vi "Create TDM.vi"() -> ()   [LabVIEW 2011]
uses:
  <vilib>/Platform/storage/lvStorage.llb/_openFunction.ctl
  <vilib>/Platform/storage/Storage.llb/usiSequenceRepresentation.ctl
  <vilib>/Platform/storage/lvStorage.llb/_defaultFilePath.vi
  <vilib>/Platform/storage/lvStorage.llb/_openStorageWithRootAutoDetect.vi
  <vilib>/Platform/storage/lvStorage.llb/xStorage/xStorageSupp/ErrorOut.vi
  <vilib>/Platform/storage/lvStorage.llb/_prepDDT.vi
  <vilib>/Platform/storage/lvStorage.llb/_createOrGetExplicitChildObject.vi
  <vilib>/Platform/storage/lvStorage.llb/_getChannelNameFromDDT.vi
  <vilib>/Platform/storage/lvStorage.llb/_createOrGetByNameExplicitChildObject.vi
  <vilib>/Platform/storage/lvStorage.llb/_saveDDT.vi
  <vilib>/Platform/storage/lvStorage.llb/_queryPropDateTime.vi
  <vilib>/Platform/storage/lvStorage.llb/_queryGenericObjects.vi
  <vilib>/Platform/storage/lvStorage.llb/_loadAllDdt.vi
  <vilib>/Platform/storage/Storage.llb/Get Object Info.vi
  <vilib>/Platform/storage/Storage.llb/__closeStorageFromObject.vi
  <vilib>/Platform/storage/lvStorage.llb/xStorage/Open Data Storage/Open Data Storage.xnode
  <vilib>/Platform/storage/lvStorage.llb/xStorage/Write Data/Write Data.xnode
  <vilib>/Platform/storage/lvStorage.llb/xStorage/Read Data/Read Data.xnode
  <vilib>/Platform/storage/lvStorage.llb/xStorage/Close Data Storage/Close Data Storage.xnode
panel:
  out "Waveform Graph":dynamicdata(graph)
  out "error out":errorcluster
  in  "stop":bool
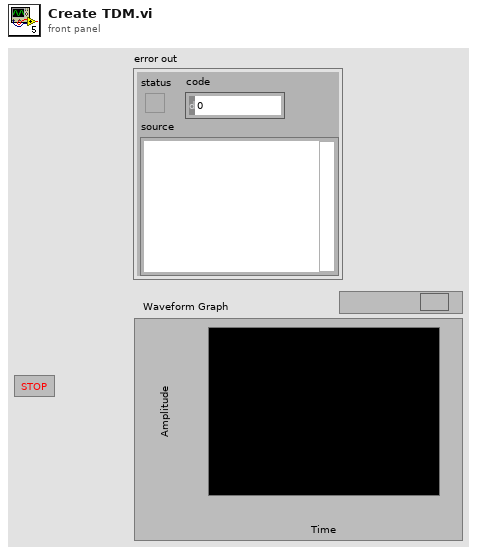
[diagram p1: front panel]
types:
  T1 = enum16{"Append values", "Replace values at index", "Replace all values"}
  T2 = enum16{"UPDATE", "READ", "QUERY", "CREATE CHILD", "CREATE", "CONNECT", "DISCONNECT"}
  T3 = typedef "usiSequenceRepresentation.ctl" = enum16{"explicit", "implicit"}
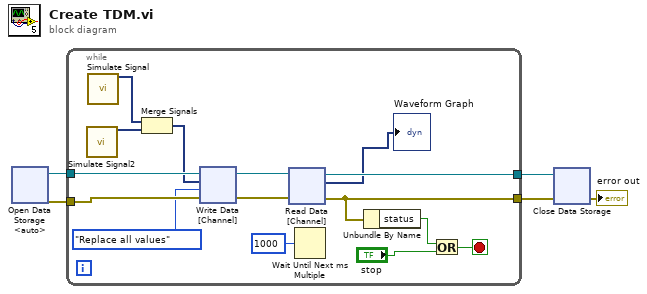
[diagram p0: block diagram]
diagram:
  n1 = xnode "Open Data Storage\n<auto>"() -> ("storage refnum (file)"=w5:refnum<k20>, "error out"=w4:errorcluster)  [unwired: 5 in, 1 out]
  n2 = while {
    tunnel: w5 -> [w20]
    tunnel: w4 -> [w19]
    tunnel: [w10] -> w3
    tunnel: [w11] -> w2
    stop <- w7 stop-if-true
    n3 = call "Simulate Signal2"() -> ("Sawtooth"=w17:dynamicdata)  [unwired: 14 in, 1 out]
    n4 = call "Simulate Signal"() -> ("Sine"=w18:dynamicdata)  [unwired: 14 in, 1 out]
    n5 = Merge Signals(w18, w17) -> (w12:dynamicdata)
    n6 = xnode "Write Data\n[Channel]"("storage refnum (file)"=w20, "error in"=w19, "Signal"=w12, "append / replace (append data values)"=T1."Replace all values") -> ("storage refnum (file) out"=w16:refnum<k20>, "error out"=w15:errorcluster)  [unwired: 1 in, 1 out]
    n7 = xnode "Read Data\n[Channel]"("storage refnum (file)"=w16, "error in"=w15) -> ("storage refnum (file) out"=w11:refnum<k20>, "error out"=w10:errorcluster, "Signal"=→"Waveform Graph":dynamicdata)  [unwired: 2 in, 1 out]
    n8 = Wait Until Next ms Multiple(millisecond multiple=u32 1000) -> ()  [unwired: 1 out]
    n9 = Unbundle By Name(w10) -> ("status"=w9:bool)
    n10 = Or(x=w9, y="stop") -> (x .or. y?=w7:bool)
  }
  n11 = xnode "Close Data Storage"("storage refnum (file)"=w2, "error in (no error)"=w3) -> ("error out"=→"error out":errorcluster)  [unwired: 1 out]
